vi "Test Error before assertion.vi"(8 "error in (no error)":errorcluster, 11 "Test Case In":refnum<class "LUnit Comparison.lvclass">) -> (0 "error out":errorcluster, 3 "Test Case Out":refnum<class "LUnit Comparison.lvclass">)   [LabVIEW 2020, in "LUnit Comparison.lvclass"]
uses:
  LUnit Comparison.lvclass
  C:/Program Files (x86)/National Instruments/LabVIEW 2020/vi.lib/Astemes/LUnit/Test Case.lvclass
  <vilib>/Astemes/LUnit/Test Case.lvclass/Test Case.ctl
  <vilib>/Astemes/LUnit/Append Fail Result.vi
  <vilib>/Astemes/LUnit/Append Pass Result.vi
  <vilib>/Astemes/LUnit/Run In UI.vi
  <vilib>/Utility/error.llb/Clear Errors.vi
  <vilib>/Astemes/LUnit/Test Case.lvclass
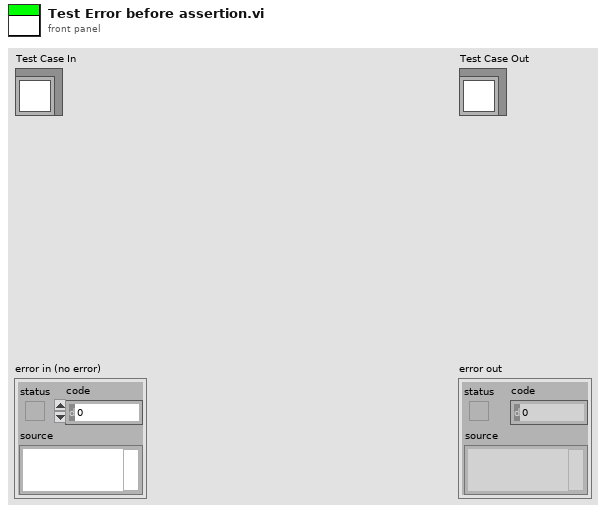
[diagram p1: front panel]
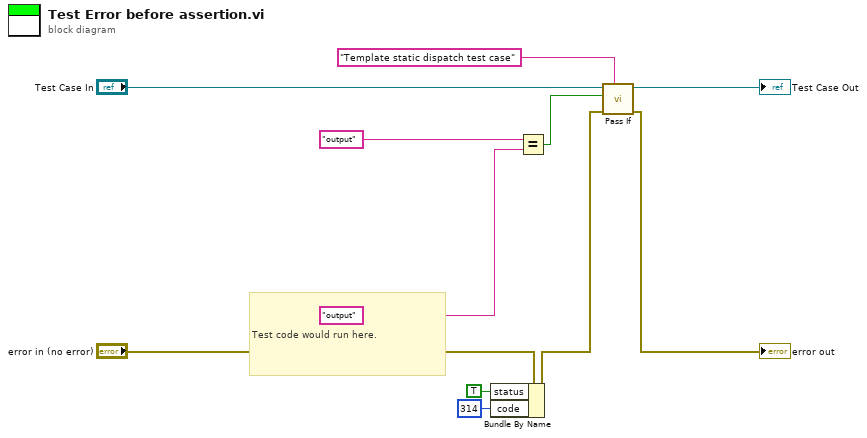
[diagram p0: block diagram]
diagram:
  # "Test code would run here."
  n1 = Bundle By Name(cluster="error in (no error)", "status"=TRUE, "code"=314) -> (w3:errorcluster)
  n2 = Equal?(x="output" ("Description"), y="output" ("Description")) -> (x = y?=w4:bool)
  n3 = call <vilib>:"Pass If.vi"("Description"="Template static dispatch test case", "error in (no error)"=w3, "Pass?"=w4, "LUnit Test Case In"="Test Case In") -> ("error out"=→"error out":errorcluster, "LUnit Test Case Out"=→"Test Case Out":refnum<class "LUnit Comparison.lvclass">)  [unwired: 6 in]
